vi "acquireValue.vi"(8 "error in (no error)":errorcluster, 10 "nextSample?":bool, 11 "settingsAppliedDomeController in":refnum<class "settingsAppliedDomeController.lvclass">) -> (0 "error out":errorcluster, 1 "function return":i32, 2 "variantData":variant, 3 "settingsAppliedDomeController out":refnum<class "settingsAppliedDomeController.lvclass">)   [LabVIEW 2016, in "SALLV_AtDome_Messaging.lvlib" / "settingsAppliedDomeController.lvclass"]
uses:
  settingsAppliedDomeController.lvclass
  ts_sallv_AtDome/SALLV_AtDome.lvlib
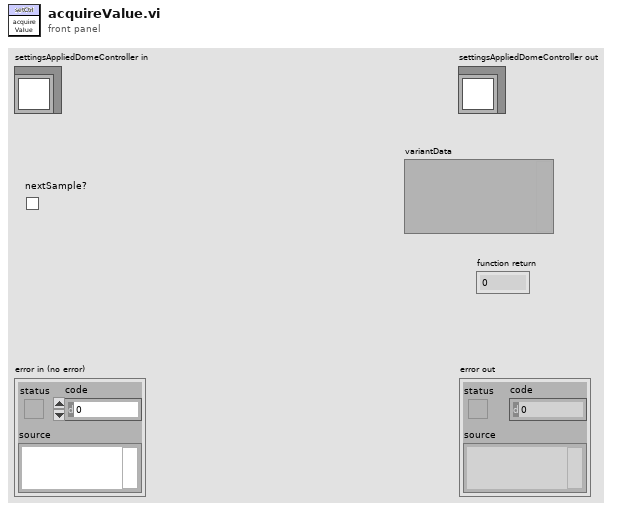
[diagram p1: front panel]
types:
  T1 = typedef "SALLV_AtDome.lvlib/logevent_settingsAppliedDomeController.ctl" = cluster{"rainSensorActivated":bool, "cloudSensorActivated":bool, "tolerance":sgl, "highSpeedDistance":sgl, "learnManual":i32, "watchdogTimer":sgl, "reversalDelay":sgl, "autoShutdownActivated":bool, "priority":i32}
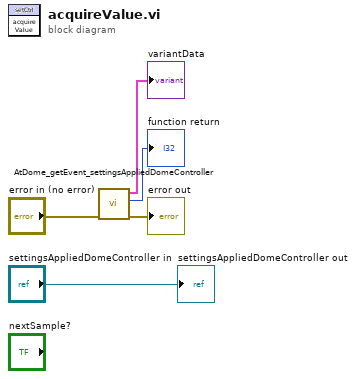
[diagram p0: block diagram]
diagram:
  n1 = call "AtDome_getEvent_settingsAppliedDomeController.vi"("error in (no error)"="error in (no error)") -> ("error out"=→"error out":errorcluster, "function return"=→"function return":i32, "logevent_settingsAppliedDomeController_Ctl out"=→"variantData":T1)  [unwired: 8 in]
  "settingsAppliedDomeController out" <- "settingsAppliedDomeController in"
